vi "Drive Teleop.vi"(9 "Joystick Buttons":bool[](array[boolean]), 11 "Joystick Axis":dbl[](array[numeric])) -> ()   [LabVIEW 2019]
uses:
  Implementation/Drive Operations.ctl
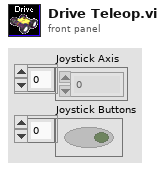
[diagram p1: front panel]
types:
  T1 = typedef "Drive Operations.ctl" = enum16{"Reserve", "Read Current", "Immediate", "Pod Racer", "Ball AA", "Feeder Station AA", "Play Back From Log"}
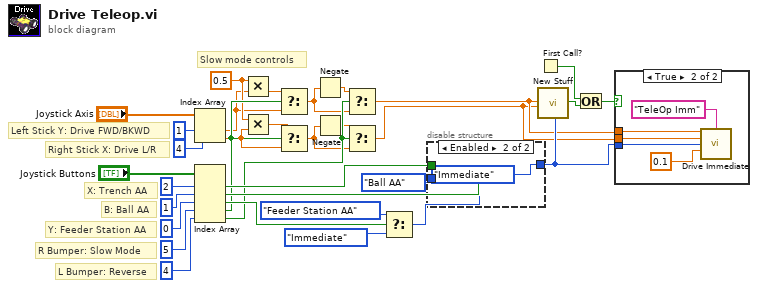
[diagram p0: block diagram]
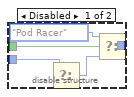
[diagram p2: hidden frame]
diagram:
  w5 = 0.5 ("x")
  # "L Bumper: Reverse"
  # "Slow mode controls"
  # "R Bumper: Slow Mode"
  # "Y: Feeder Station AA"
  # "B: Ball AA"
  # "X: Trench AA"
  # "Right Stick X: Drive L/R"
  # "Left Stick Y: Drive FWD/BKWD"
  n1 = Index Array(array="Joystick Axis", index #1=1 ("index"), index #2=4 ("index")) -> (element #1=w4:dbl, element #2=w14:dbl)
  n2 = Index Array(array="Joystick Buttons", index #1=2 ("index"), index #2=1 ("index"), index #3=0 ("index"), index #4=5 ("index"), index #5=4 ("index")) -> (element #1=w27:bool, element #2=w25:bool, element #3=w21:bool, element #4=w17:bool, element #5=w12:bool)
  n3 = Multiply(x=w5, y=w4) -> (x*y=w16:dbl)
  n4 = Multiply(x=w5, y=w14) -> (x*y=w15:dbl)
  n5 = Select(t=w16, s=w17, f=w4) -> (s? t:f=w11:dbl)
  n6 = Select(t=w15, s=w17, f=w14) -> (s? t:f=w8:dbl)
  n7 = Negate(x=w11) -> (-x=w10:dbl)
  n8 = Negate(x=w8) -> (-x=w9:dbl)
  n9 = Select(t=w10, s=w12, f=w11) -> (s? t:f=w7:dbl)
  n10 = Select(t=w9, s=w12, f=w8) -> (s? t:f=w6:dbl)
  n11 = Select(t=Drive_Operations."Feeder Station AA" ("Operation"), s=w21, f=Drive_Operations."Immediate" ("Operation")) -> (s? t:f=w23:T1)
  n12 = disable-structure shown="Enabled" {
    disable-tunnel: Drive_Operations."Ball AA" ("Operation") -> [w40 _]
    disable-tunnel: [w37 Drive_Operations."Immediate" ("Operation")] -> w28
    disable-tunnel: w27 -> [w36 _]
    disable-tunnel: w25 -> [w35 _]
    disable-tunnel: w23 -> [w34 _]
    frame Disabled {
      n13 = Select(t=w40, s=w35, f=w34) -> (s? t:f=w39:T1)
      n14 = Select(t=Drive_Operations."Pod Racer" ("Operation"), s=w36, f=w39) -> (s? t:f=w37:T1)
    }
    frame Enabled {
    }
  }
  n15 = First Call?() -> (First Call?: T/F=w1:bool)
  n16 = call "New Stuff.vi"("Variant 3"=w7, "Variant 16"=w6, "Variant 9"=w28) -> ("x != y?"=w2:bool)  [unwired: 24 in]
  n17 = Or(x=w1, y=w2) -> (x .or. y?=w3:bool)
  n18 = case shown="True" w3 {
    tunnel: w28 -> [_ w45]
    tunnel: w7 -> [_ w43]
    tunnel: w6 -> [_ w42]
    frame False {
    }
    frame True {
      n19 = call "Drive Immediate.vi"("Fowards/Backwards"=w43, "Description"="TeleOp Imm", "Turning"=w42, "Operation"=w45, "Deadband Value"=0.1) -> ()  [unwired: 10 in, 1 out]
    }
  }
